vi "CIMAQ_SoftTruncate.vi"(7 "Cutoff (%)":dbl, 10 "Image Dst":T1, 11 "Image Src":T1) -> (3 "Image":T1(plugin-control))   [LabVIEW 2017]
uses:
  <vilib>/vision/Image Controls.llb/IMAQ Image.ctl
  <vilib>/Analysis/baseanly.llb/Quick Scale 2D.vi
  <vilib>/vision/NI_Vision_Development_Module.lvlib
  <vilib>/Analysis/NI_AALBase.lvlib
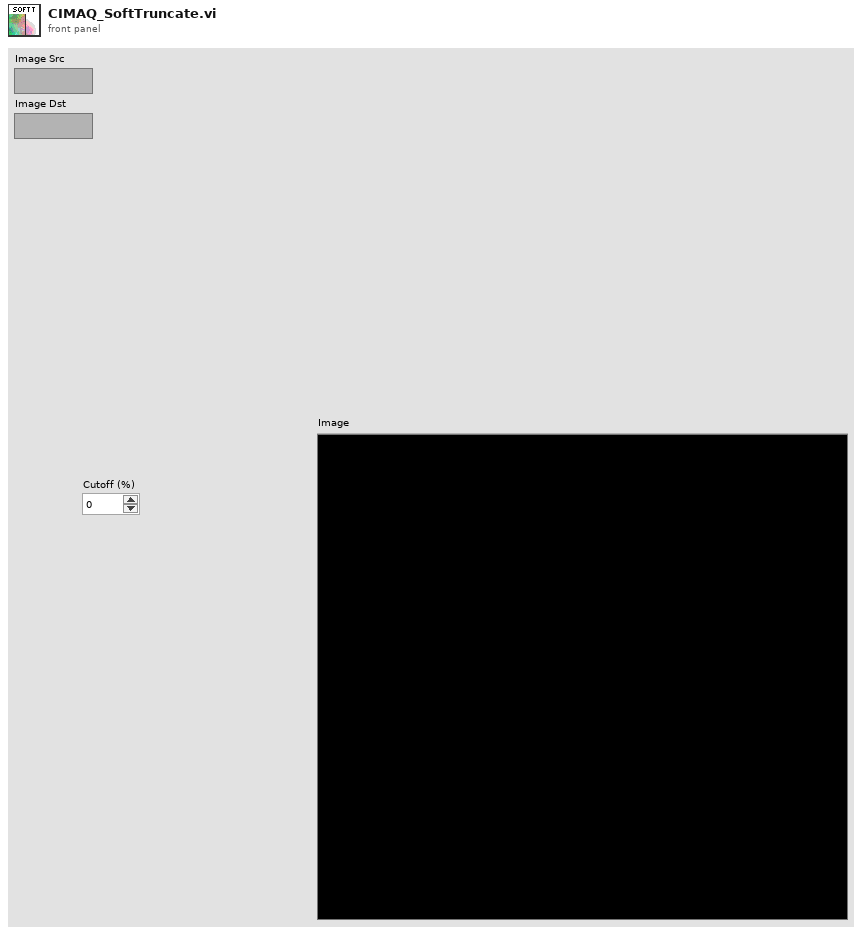
[diagram p1: front panel]
types:
  T1 = typedef "IMAQ Image.ctl" = refnum<image>
  T2 = typedef "Image Type" = u32
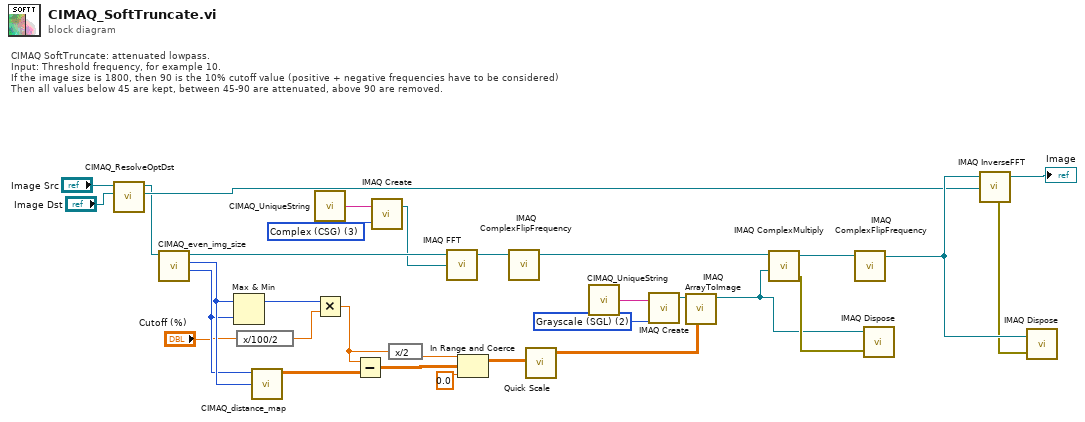
[diagram p0: block diagram]
diagram:
  w19 = T2 2 items=["Grayscale (U8)", "Grayscale (I16)", "Grayscale (SGL)", "Complex (CSG)", "RGB (U32)", "HSL (U32)", "RGB (U64)", "Grayscale (U16)"] ("Image Type")
  w26 = T2 3 items=["Grayscale (U8)", "Grayscale (I16)", "Grayscale (SGL)", "Complex (CSG)", "RGB (U32)", "HSL (U32)", "RGB (U64)", "Grayscale (U16)"] ("Image Type")
  # "CIMAQ SoftTruncate: attenuated lowpass.\nInput: Threshold frequency, for example 10. \nIf the image size is 1800, then 90 is the 10% cutoff value (positive + negative frequencies have to be considered)\nThen all values below 45 are kept, between 45-90 are attenuated, above 90 are removed."
  n1 = call <userlib>:"CIMAQ_ResolveOptDst.vi"("Dst(optional)"="Image Dst", "Src"="Image Src") -> ("Dst"=w3:T1, "Src"=w1:T1)  [unwired: 7 in]
  n2 = call <userlib>:"CIMAQ_even_img_size.vi"("img"=w1) -> ("resolution_y"=w23:u32, "resolution_x"=w24:u32, "img"=w31:T1)  [unwired: 8 in]
  n3 = Max & Min(x=w24, y=w23) -> (max(x,y)=w21:u32)  [unwired: 1 out]
  n4 = expression code="x/100/2"("Cutoff (%)") -> (w22:dbl)
  n5 = call <userlib>:"CIMAQ_distance_map.vi"("size_x"=w24, "size_y"=w23) -> ("distance_map"=w15:dbl[][])  [unwired: 9 in]
  n6 = call <userlib>:"CIMAQ_UniqueString.vi"() -> ("String"=w10:string)  [unwired: 5 in]
  n7 = Multiply(x=w21, y=w22) -> (x*y=w14:dbl)
  n8 = Subtract(x=w14, y=w15) -> (x-y=w13:dbl[][])
  n9 = call "IMAQ Create"("Image Name"=w10, "Image Type"=w26) -> ("New Image"=w25:T1)  [unwired: 3 in, 1 out]
  n10 = expression code="x/2"(w14) -> (w16:dbl)
  n11 = call "IMAQ FFT"("Image Dst"=w25, "Image Src"=w31) -> ("Image Dst Out"=w30:T1)  [unwired: 2 in, 1 out]
  n12 = In Range and Coerce(upper limit=w16, x=w13, lower limit=0.0 ("x*y")) -> (coerced(x)=w12:dbl[][])  [unwired: 1 out]
  n13 = call "IMAQ ComplexFlipFrequency"("Image Src"=w30) -> ("Image Dst Out"=w29:T1)  [unwired: 3 in, 1 out]
  n14 = call-poly <vilib>:"Quick Scale.vi"("X"=w12) -> ("Yij=Xij/Max|X|"=w11:dbl[][])  [unwired: 2 out]
  n15 = call <userlib>:"CIMAQ_UniqueString.vi"() -> ("String"=w9:string)  [unwired: 5 in]
  n16 = call "IMAQ Create"("Image Name"=w9, "Image Type"=w19) -> ("New Image"=w28:T1)  [unwired: 3 in, 1 out]
  n17 = call "IMAQ ArrayToImage"("Image Pixels (Float)"=w11, "Image"=w28) -> ("Image Out"=w7:T1)  [unwired: 8 in, 1 out]
  n18 = call "IMAQ ComplexMultiply"("Image Src A"=w29, "Image Src B"=w7) -> ("Image Dst Out"=w27:T1, "error out"=w8:errorcluster)  [unwired: 5 in]
  n19 = call "IMAQ ComplexFlipFrequency"("Image Src"=w27) -> ("Image Dst Out"=w6:T1)  [unwired: 3 in, 1 out]
  n20 = call "IMAQ Dispose"("Image"=w7, "error in (no error)"=w8) -> ()  [unwired: 4 in, 1 out]
  n21 = call "IMAQ InverseFFT"("Image Dst"=w3, "Image Src"=w6) -> ("error out"=w5:errorcluster, "Image Dst Out"=→"Image":T1)  [unwired: 2 in]
  n22 = call "IMAQ Dispose"("Image"=w6, "error in (no error)"=w5) -> ()  [unwired: 4 in, 1 out]
